vi "setCategoryDefaultAmount.vi"(8 "error in (no error)":errorcluster, 9 "Default Amount":dbl, 10 "Name":string, 11 "Account History in":refnum<class "Account History.lvclass">) -> (0 "error out":errorcluster, 3 "Account History out":refnum<class "Account History.lvclass">)   [LabVIEW 2018, in "Account History.lvclass"]
uses:
  Account History.lvclass
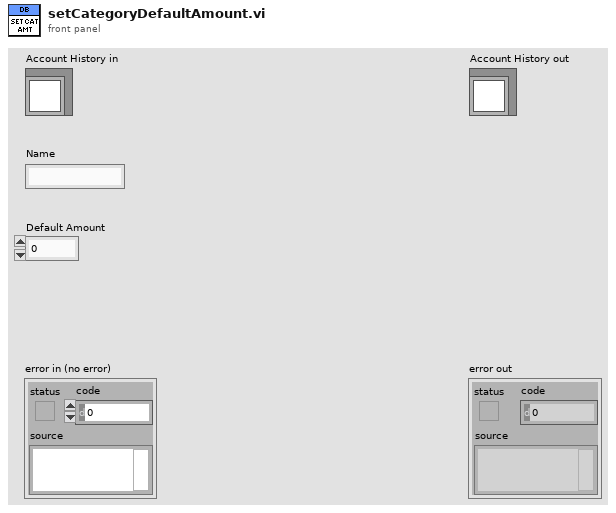
[diagram p1: front panel]
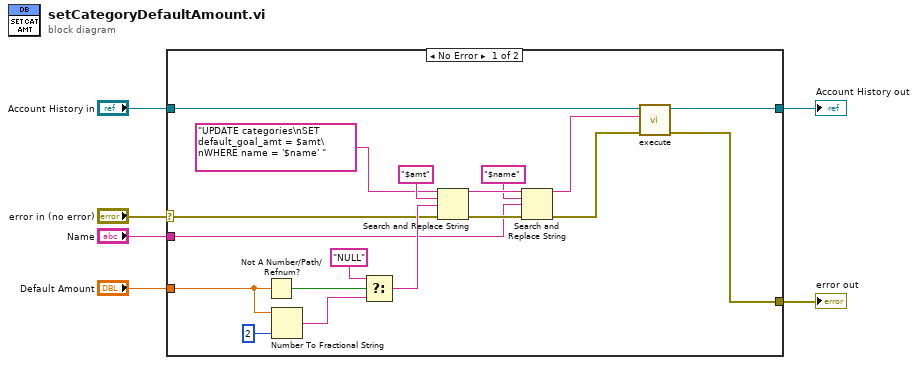
[diagram p0: block diagram]
diagram:
  n1 = case shown="No Error" "error in (no error)" {
    selector: "error in (no error)" -> [w11 w26]
    tunnel: [w22 w26] -> w5
    tunnel: [w23 w25] -> w3
    tunnel: "Account History in" -> [w24 w25]
    tunnel: "Default Amount" -> [w10 _]
    tunnel: "Name" -> [w9 _]
    frame No Error {
      n2 = Not A Number/Path/Refnum?(number/path/refnum=w10) -> (NaN/Path/Refnum?=w15:bool)
      n3 = Number To Fractional String(number=w10, precision (6)=i16 2) -> (F-format string=w14:string)  [unwired: 2 in]
      n4 = Select(t="NULL" ("search string"), s=w15, f=w14) -> (s? t:f=w13:string)
      n5 = Search and Replace String(input string="UPDATE categories\nSET default_goal_amt = $amt\nWHERE name = '$name' ", search string="$amt", replace string=w13, error in=w11) -> (result string=w19:string, error out=w20:errorcluster)  [unwired: 4 in, 2 out]
      n6 = Search and Replace String(input string=w19, search string="$name", replace string=w9, error in=w20) -> (result string=w7:string, error out=w8:errorcluster)  [unwired: 4 in, 2 out]
      n7 = call "execute.vi"("error in (no error)"=w8, "SQL query"=w7, "Database in"=w24) -> ("error out"=w22:errorcluster, "Database out"=w23:refnum<class "Account History.lvclass">)  [unwired: 7 in]
    }
    frame Error {
    }
  }
  "error out" <- w5
  "Account History out" <- w3
